vi "main.vi"() -> ()   [LabVIEW 2021]
uses:
  source/system/system.lvclass
  source/system.threading/system.threading.lvclass
  source/system.logging/system.logging.lvclass
panel:
  out "exit_code":errorcluster
  in  "Abort":bool
  # "main application entry point, this is a general container for the application layout"
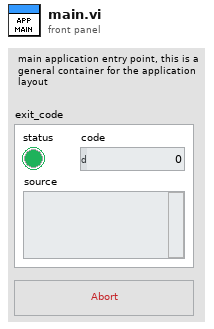
[diagram p1: front panel]
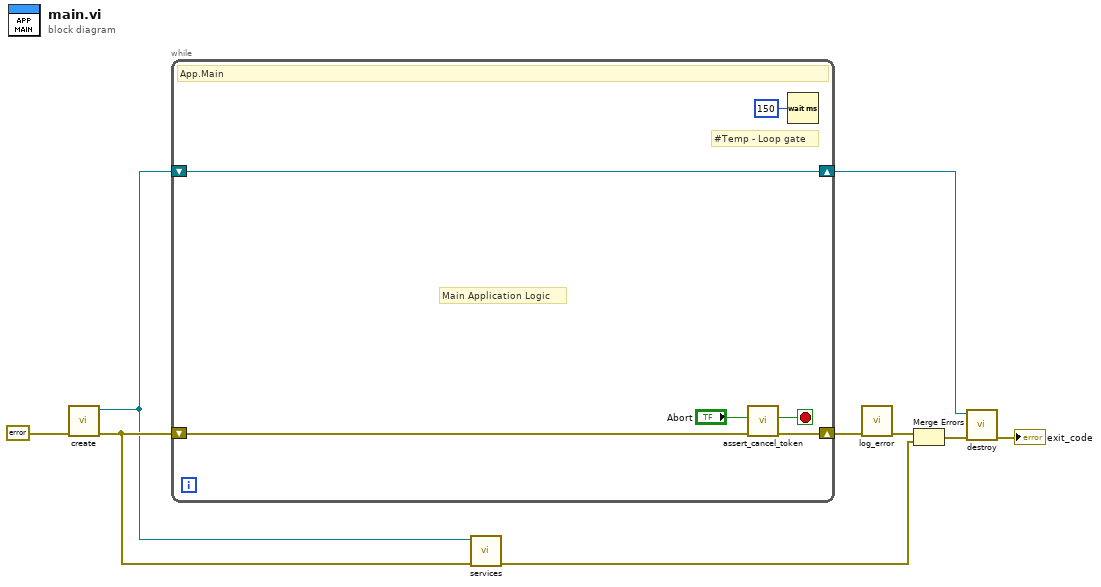
[diagram p0: block diagram]
diagram:
  n1 = call "create.vi"("error in (no error)"=errorcluster {"status"=FALSE, "code"=0, "source"=""}) -> ("error out"=w5:errorcluster, "system out"=w4:refnum<class "system.lvclass">)  [unwired: 9 in]
  n2 = while "MainThread" {
    shift-right: [w10] -> w2
    shift-left: w5 -> [w11]
    shift-right: [w14] -> w8
    shift-left: w4 -> [w14]
    stop <- w12 stop-if-true
    # "Main Application Logic"
    # "#Temp - Loop gate"
    # "App.Main"
    n3 = call "assert_cancel_token.vi"("error in (no error)"=w11, "abort_in"="Abort") -> ("error out"=w10:errorcluster, "abort_out"=w12:bool)  [unwired: 8 in]
    n4 = Wait (ms)(milliseconds to wait=u32 150) -> ()  [unwired: 1 out]
  }
  n5 = call "services.vi"("error in (no error)"=w5, "system in"=w4) -> ("error out"=w3:errorcluster)  [unwired: 9 in]
  n6 = call "log_error.vi"("error in (no error)"=w2) -> ("error out"=w1:errorcluster)  [unwired: 10 in]
  n7 = Merge Errors(w1, w3) -> (w6:errorcluster)
  n8 = call "destroy.vi"("error in (no error)"=w6, "system in"=w8) -> ("error out"=→"exit_code":errorcluster)  [unwired: 9 in]
